vi "Fault_ID_Parse.vi"(8 "Enum":enum16{"Sequence", "Table"}(ring), 11 "Numeric":u32) -> (3 "String":string)   [LabVIEW 2016]
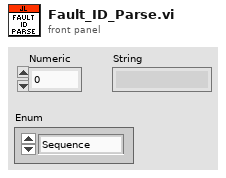
[diagram p1: front panel]
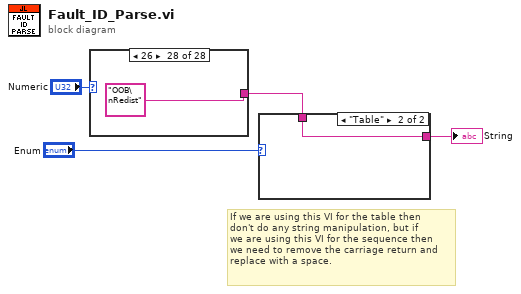
[diagram p0: block diagram]
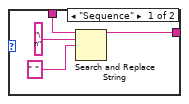
[diagram p2: hidden frame]
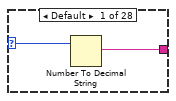
[diagram p3: hidden frame]
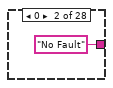
[diagram p4: hidden frame]
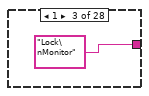
[diagram p5: hidden frame]
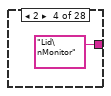
[diagram p6: hidden frame]
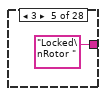
[diagram p7: hidden frame]
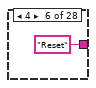
[diagram p8: hidden frame]
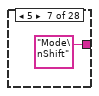
[diagram p9: hidden frame]
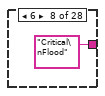
[diagram p10: hidden frame]
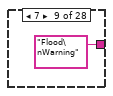
[diagram p11: hidden frame]
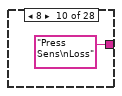
[diagram p12: hidden frame]
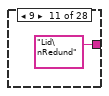
[diagram p13: hidden frame]
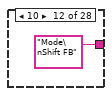
[diagram p14: hidden frame]
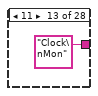
[diagram p15: hidden frame]
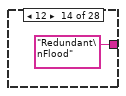
[diagram p16: hidden frame]
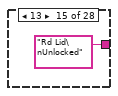
[diagram p17: hidden frame]
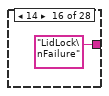
[diagram p18: hidden frame]
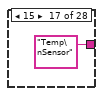
[diagram p19: hidden frame]
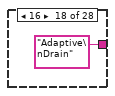
[diagram p20: hidden frame]
diagram:
  # "If we are using this VI for the table then\ndon't do any string manipulation, but if\nwe are using this VI for the sequence then\nwe need to remove the carriage return and\nreplace with a space."
  n1 = case shown="26" "Numeric" {
    selector: "Numeric" -> [w6 _ _ _ _ _ _ _ _ _ _ _ _ _ _ _ _ _ _ _ _ _ _ _ _ _ _ _]
    tunnel: [w5 "No Fault" "Lock\nMonitor" "Lid\nMonitor" "Locked\nRotor " "Reset" "Mode\nShift" "Critical\nFlood" "Flood\nWarning" "Press Sens\nLoss" "Lid\nRedund" "Mode\nShift FB" "Clock\nMon" "Redundant\nFlood" "Rd Lid\nUnlocked" "LidLock\nFailure" "Temp\nSensor" "Adaptive\nDrain" "Dry Load\nTO" "Drain\nClearing" "UI State\nTimeout" "Crit\nFlood Gal" "Flood\nWarn Gal" "OOB\nDryLoad" "Crit\nLid Lock" "Lid\n Logic" "Press Sens\nDropout" "OOB\nRedist"] -> w3
    frame Default {
      n2 = Number To Decimal String(number=w6) -> (decimal integer string=w5:string)  [unwired: 1 in]
    }
    frame 0 {
    }
    frame 1 {
    }
    frame 2 {
    }
    frame 3 {
    }
    frame 4 {
    }
    frame 5 {
    }
    frame 6 {
    }
    frame 7 {
    }
    frame 8 {
    }
    frame 9 {
    }
    frame 10 {
    }
    frame 11 {
    }
    frame 12 {
    }
    frame 13 {
    }
    frame 14 {
    }
    frame 15 {
    }
    frame 16 {
    }
    frame 17 {
    }
    frame 18 {
    }
    frame 19 {
    }
    frame 20 {
    }
    frame 21 {
    }
    frame 22 {
    }
    frame 23 {
    }
    frame 24 {
    }
    frame 25 {
    }
    frame 26 {
    }
  }
  n3 = case shown="\"Table\"" "Enum" {
    tunnel: w3 -> [w37 w38]
    tunnel: [w34 w38] -> w2
    frame "Sequence" {
      n4 = Search and Replace String(input string=w37, search string="\n", replace string=" " ("replace string (\"\")")) -> (result string=w34:string)  [unwired: 5 in, 3 out]
    }
    frame "Table" {
    }
  }
  "String" <- w2
